vi "Add Configuration Files Section.vi"(8 "error in":errorcluster, 11 "custom device":T1 format="%.0x") -> (0 "error out":errorcluster, 2 "configuration files section":T1 format="%.0x", 3 "custom device out":T1 format="%.0x")   [LabVIEW 2020, in "AIM MIL-STD-1553 Scripting.lvlib"]
doc: "Adds the <b>configuration file section</b> to the custom device."
uses:
  AIM MIL-STD-1553 Scripting.lvlib
  <vilib>/NI VeriStand/Custom Device API/Custom Device Item Ref.ctl
  Constants.vi
  <vilib>/NI VeriStand/Custom Device API/Custom Device API.lvlib
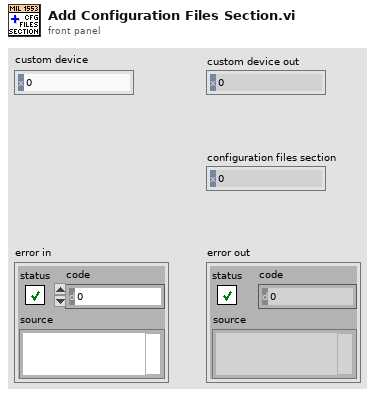
[diagram p1: front panel]
types:
  T1 = typedef "Custom Device API.lvlib/Custom Device Item Ref.ctl" = u64
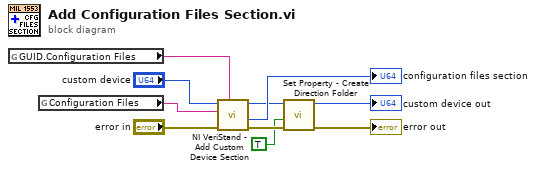
[diagram p0: block diagram]
diagram:
  n1 = global read "Constants.vi" "GUID.Configuration Files"() -> (w7:string)
  n2 = global read "Constants.vi" "Configuration Files"() -> (w6:string)
  n3 = call <vilib>:"NI VeriStand - Add Custom Device Section.vi"("GUID (Default Section)"=w7, "error in (no error)"="error in", "Section Name"=w6, "Parent Ref in"="custom device") -> ("error out"=w3:errorcluster, "Section Ptr"=→"configuration files section":T1, "Parent Ref out"=w5:T1)  [unwired: 4 in, 1 out]
  n4 = call "Set Property - Create Direction Folder.vi"("error in"=w3, "create Tx/Rx folders for subaddresses?"=TRUE, "custom device"=w5) -> ("error out"=→"error out":errorcluster, "custom device out"=→"custom device out":T1)  [unwired: 7 in]
